vi "Unsubscribe (async) JSON.vi"(7 "Options":string="{}", 8 "error in (no error)":errorcluster, 10 "Topic":string, 11 "WAMP Client in":refnum<class "WAMP Client.lvclass">) -> (0 "error out":errorcluster, 2 "notifier out":refnum<notifier>, 3 "WAMP Client out":refnum<class "WAMP Client.lvclass">)   [LabVIEW 2020, in "wamplv.lvlib" / "WAMP Client.lvclass"]
uses:
  WAMP Client.lvclass
  TypeDef/UNSUBSCRIBE Request Data (JSON).ctl
  wamplv.lvlib
  Private/Requests/Unsubscribe/Unsubscribe JSON/Unsubscribe JSON.lvclass
  Private/Message loop classes/ErrorOrSuccess JSON/ErrorOrSuccess JSON.lvclass
  C:/local/wamplv/Private/Requests/IGenericWithOutputInternalMessage/IGenericWithOutputInternalMessage/IGenericWithOutputInternalMessage.lvclass
  C:/local/wamplv/Private/Requests/IInternalMessage/IInternalMessage.lvclass
  C:/local/wamplv/Private/Requests/Unsubscribe/IUnsubscribe/IUnsubscribe.lvclass
  C:/local/wamplv/Private/Requests/IContainersNotiferOrEvents/IContainersNotiferOrEvents.lvclass
  C:/local/wamplv/Private/Requests/Unsubscribe/Unsubscribe JSON/Unsubscribe JSON.lvclass
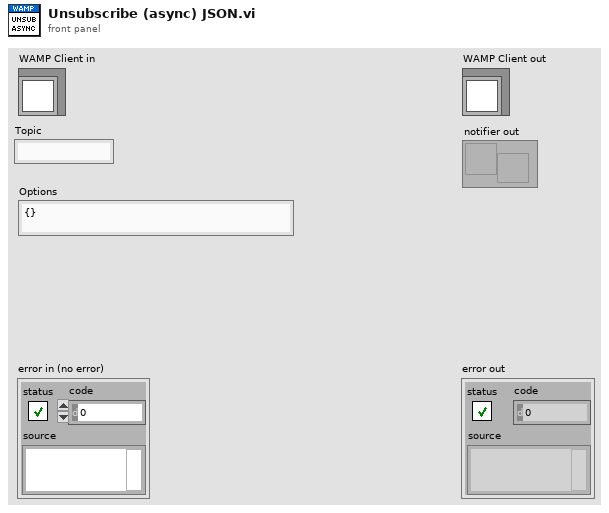
[diagram p1: front panel]
types:
  T1 = typedef "wamplv.lvlib/UNSUBSCRIBE Request Data (JSON).ctl" = cluster{"Topic":string, "Options":string, "Result notifier out":refnum<notifier>}
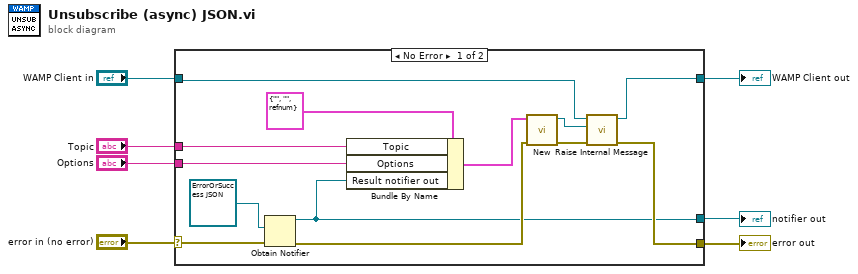
[diagram p0: block diagram]
diagram:
  n1 = case shown="No Error" "error in (no error)" {
    selector: "error in (no error)" -> [w17 w22]
    tunnel: [w10 w22] -> w6
    tunnel: [w13 w21] -> w4
    tunnel: "WAMP Client in" -> [w20 w21]
    tunnel: "Topic" -> [w19 _]
    tunnel: [w8 _] -> w1
    tunnel: "Options" -> [w16 _]
    frame No Error {
      n2 = Obtain Notifier(notification data type=refnum<class "ErrorOrSuccess JSON.lvclass"> refnum ("wamplv.lvlib:ErrorOrSuccess JSON.lvclass"), error in (no error)=w17) -> (notifier out=w8:refnum<notifier>, error out=w14:errorcluster)  [unwired: 2 in, 1 out]
      n3 = Bundle By Name(cluster=T1 {"Topic"="", "Options"="", "Result notifier out"=refnum} ("Cluster"), "Topic"=w19, "Options"=w16, "Result notifier out"=w8) -> (w15:T1)
      n4 = call "New.vi"("error in (no error)"=w14, "UNSUBSCRIBE Request Data (JSON)"=w15) -> ("error out"=w12:errorcluster, "Unsubscribe JSON out"=w11:refnum<class "Unsubscribe JSON.lvclass">)  [unwired: 8 in]
      n5 = call "Raise Internal Message.vi"("error in (no error)"=w12, "IInternalMessage"=w11, "WAMP Client in"=w20) -> ("error out"=w10:errorcluster, "WAMP Client out"=w13:refnum<class "WAMP Client.lvclass">)  [unwired: 7 in]
    }
    frame Error {
    }
  }
  "error out" <- w6
  "WAMP Client out" <- w4
  "notifier out" <- w1
